vi "ReadPixelRgbaU32.vi"(8 "error in":errorcluster, 9 "Y Coordinate":i32, 10 "X Coordinate":i32, 11 "Image Reference In":T2) -> (0 "error out":errorcluster, 2 "Pixel value":T1, 3 "Image Reference Out":T2)   [LabVIEW 2024, in "OpenLvVision_Image.lvlib" / "DataAccess.lvlib"]
doc: "Provides the pixel's value at the given coordinates."
uses:
  DataAccess.lvlib
  Management/TypeDef/Image.ctl
  TypeDef/RgbaU32.ctl
  <vilib>/Utility/error.llb/Error Cluster From Error Code.vi
  <vilib>/ErrorRing/Error Ring.xnode
  Management/Management.lvlib
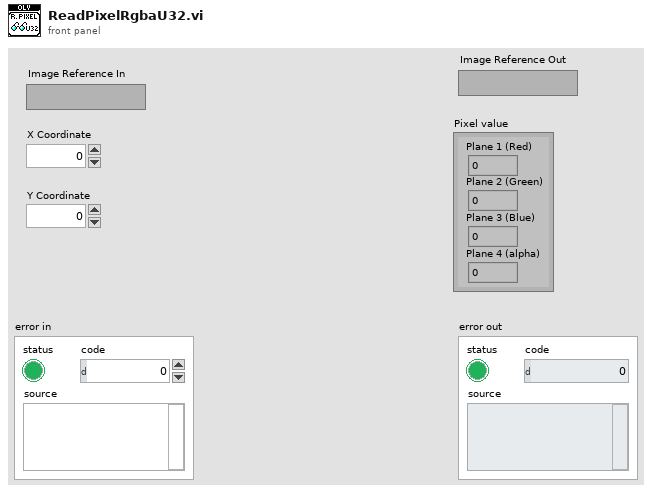
[diagram p1: front panel]
types:
  T1 = typedef "OpenLvVision_Image.lvlib/DataAccess.lvlib/RgbaU32.ctl" = cluster{"Plane 1 (Red)":u8, "Plane 2 (Green)":u8, "Plane 3 (Blue)":u8, "Plane 4 (alpha)":u8}
  T2 = typedef "OpenLvVision_Image.lvlib/Management.lvlib/Image.ctl" = refnum<image>
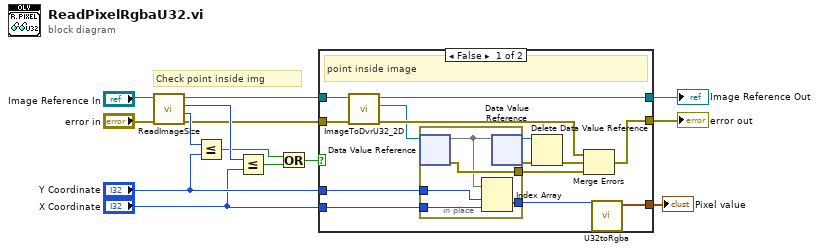
[diagram p0: block diagram]
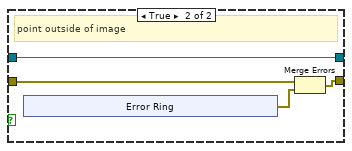
[diagram p2: hidden frame]
diagram:
  # "Check point inside img"
  n1 = call "ReadImageSize.vi"("error in"="error in", "Image Reference In"="Image Reference In") -> ("error out"=w4:errorcluster, "Height"=w10:i32, "Width"=w12:i32, "Image Reference Out"=w11:T2)  [unwired: 6 in]
  n2 = Less Or Equal?(x=w10, y="Y Coordinate") -> (x <= y?=w8:bool)
  n3 = Less Or Equal?(x=w12, y="X Coordinate") -> (x <= y?=w9:bool)
  n4 = Or(x=w8, y=w9) -> (x .or. y?=w7:bool)
  n5 = case shown="False" w7 {
    tunnel: w11 -> [w28 w35]
    tunnel: w4 -> [w27 w37]
    tunnel: "Y Coordinate" -> [w19 _]
    tunnel: "X Coordinate" -> [w18 _]
    tunnel: [w26 w35] -> w3
    tunnel: [w17 w34] -> w2
    tunnel: [w15 _] -> w1
    frame False {
      # "point inside image"
      n6 = call "ImageToDvrU32_2D.vi"("error in"=w27, "Image Reference In"=w28) -> ("error out"=w21:errorcluster, "EDVR 2D U32"=w20:refnum<data-value>, "Image Reference Out"=w26:T2)  [unwired: 6 in, 1 out]
      n7 = in-place {
        in-place-border: [w33] -> w24
        in-place-border: w19 -> [w31]
        in-place-border: w18 -> [w30]
        in-place-border: [w29] -> w16
        n8 = in-place-dvr #1(w20) -> (w32:u32[][], w33:errorcluster)
        n9 = Index Array(array=w32, index (row)=w31, index (col)=w30) -> (element=w29:u32)
        n10 = in-place-dvr #1(w32) -> (w22:refnum<data-value>, w23:errorcluster)
      }
      n11 = Delete Data Value Reference(data value reference=w22, error in=w23) -> (error out=w25:errorcluster)  [unwired: 1 out]
      n12 = Merge Errors(w21, w25, w24) -> (w17:errorcluster)
      n13 = call "U32toRgba.vi"("U32"=w16) -> ("Rgba"=w15:T1)  [unwired: 10 in]
    }
    frame True {
      # "point outside of image"
      n14 = xnode "Error Ring"() -> ("error out"=w36:errorcluster)
      n15 = Merge Errors(w37, w36) -> (w34:errorcluster)
    }
  }
  "error out" <- w2
  "Image Reference Out" <- w3
  "Pixel value" <- w1
